vi "Extended Kalman Filter (GPS & IMU Fusion) 수정중(H=eye(4)로).vi"(0 "R (v의 공분산행렬_측정잡음)_모델링필요":dbl[][](array[numeric])=[[100000000.0, 0.0, 0.0, 0.0], [0.0, 100000000.0, 0.0, 0.0], [0.0, 0.0, 100000.0, 0.0], [0.0, 0.0, 0.0, 10.0]], 4 "Q (w의 공분산행렬_시스템잡음)_모델링필요":dbl[][](array[numeric])=[[50000.0, 0.0, 0.0, 0.0], [0.0, 50000.0, 0.0, 0.0], [0.0, 0.0, 0.001, 0.0], [0.0, 0.0, 0.0, 0.01]], 5 "theta_IMU":dbl, 6 "dt (측정주기)":dbl=0.02, 7 "v_Encoder":dbl, 10 "X_GPS Raw":dbl[](array[numeric])) -> (2 "X_EKF":dbl[](array[numeric]))   [LabVIEW 2016]
uses:
  <vilib>/imath/engines/lvmath2/RunTimeEngine/IndexRead/NIMS M(S).vi
  <instcachedir>/0/NIMS M(S)_B826C018497E4940AE96BD27B540B6FB.lvgen/NIMS M(S)_B826C018497E4940AE96BD27B540B6FB_000.vi
  <vilib>/imathl/engines/lvmath/Functions/Error Handling/Create Error.vi
  <vilib>/imath/engines/lvmath2/RunTimeEngine/BuiltInFunctions/deg_to_rad/NIMS_deg_to_rad.vi
  <instcachedir>/0/NIMS_deg_to_rad_4A81D684CE8D4DD79924F5AB74D756E1.lvgen/NIMS_deg_to_rad_4A81D684CE8D4DD79924F5AB74D756E1_001.vi
  <vilib>/imath/engines/lvmath2/RunTimeEngine/ArithmeticOperatorToken/NIMS_ArithmeticOperator_multmx.vi
  <instcachedir>/0/NIMS_ArithmeticOperator_multmx_4A56FE5C615140CE835D4DB5891BF065.lvgen/NIMS_ArithmeticOperator_multmx_4A56FE5C615140CE835D4DB5891BF065_004.vi
  <vilib>/imath/engines/lvmath2/RunTimeEngine/ArithmeticOperatorToken/NIMS_ArithmeticOperator_plus.vi
  <instcachedir>/0/NIMS_ArithmeticOperator_plus_0120E0498A0F4B4B9BDCAC2554767A4E.lvgen/NIMS_ArithmeticOperator_plus_0120E0498A0F4B4B9BDCAC2554767A4E_003.vi
  <vilib>/imath/engines/lvmath2/RunTimeEngine/ErrorHandling/NIMS_Create Error From Enums.vi
  <vilib>/imath/engines/lvmath2/RunTimeEngine/BuiltInFunctions/inv/NIMS_inv(GM).vi
  <instcachedir>/0/NIMS_inv(GM)_A6DF8FE880224208AACFE4CF9F659502.lvgen/NIMS_inv(GM)_A6DF8FE880224208AACFE4CF9F659502_000.vi
  <vilib>/imath/engines/lvmath2/RunTimeEngine/ArithmeticOperatorToken/NIMS_ArithmeticOperator_multmx(M,CV).vi
  <instcachedir>/0/NIMS_ArithmeticOperator_multmx(M,CV)_EE734FC8520844C9A7CC1A67008668A3.lvgen/NIMS_ArithmeticOperator_multmx(M,CV)_EE734FC8520844C9A7CC1A67008668A3_000.vi
  <vilib>/imath/engines/lvmath2/RunTimeEngine/ArithmeticOperatorToken/NIMS_ArithmeticOperator_minus.vi
  <instcachedir>/0/NIMS_ArithmeticOperator_minus_E3B65B1D26A44BB184AFDC5B3F458E3D.lvgen/NIMS_ArithmeticOperator_minus_E3B65B1D26A44BB184AFDC5B3F458E3D_002.vi
  <vilib>/imath/engines/lvmath2/RunTimeEngine/NodeEndStatement/NIMS_NodeEndStatement_Output.vi
  <instcachedir>/0/NIMS_NodeEndStatement_Output_53EC0D466D134D7ABD903AC30B43404B.lvgen/NIMS_NodeEndStatement_Output_53EC0D466D134D7ABD903AC30B43404B_002.vi
  <vilib>/imath/engines/lvmath2/RunTimeEngine/ErrorHandling/NIMS_Finalize Error.vi
panel:
  out "P (Covariance Matrix))":dbl[][](array[numeric])
  out "K (Kalman Gain)":dbl[][](array[numeric])
  in  "P0 (공분산 행렬 초기값)_모델링필요":dbl[][](array[numeric])=[[1.0, 0.0, 0.0, 0.0], [0.0, 1.0, 0.0, 0.0], [0.0, 0.0, 1.0, 0.0], [0.0, 0.0, 0.0, 1.0]]
  # "GPS 측정값\n \n  GPS Input = [ x_Nav  y_Nav  h  theta_GPS ]'\n\n      x_Nav : 항법좌표계로 변환한 X좌표\n\n      y_Nav : 항법좌표계로 변환한 Y좌표\n\n      theta_GPS : 방향각 (Heading angle)\n\n      v_GPS: 차량의 속도 (Speed)"
  # "X(State)= [ x y theta v ]'"
  # "IMU & Encoder 측정값\n\n       theta_IMU : 방향각 (yaw angle)\n\n       v_Encoder : 차량의 속도 (Speed)"
  # "모델링 필요\n\n1, X0:   상태변수 초기값\n2. dt:    측정시간 (Hz)\n2. P0:   공분산행렬 초기값\n3. Q:    시스템노이즈 공분산행렬\n4. R:     측정노이즈 공분산행렬"
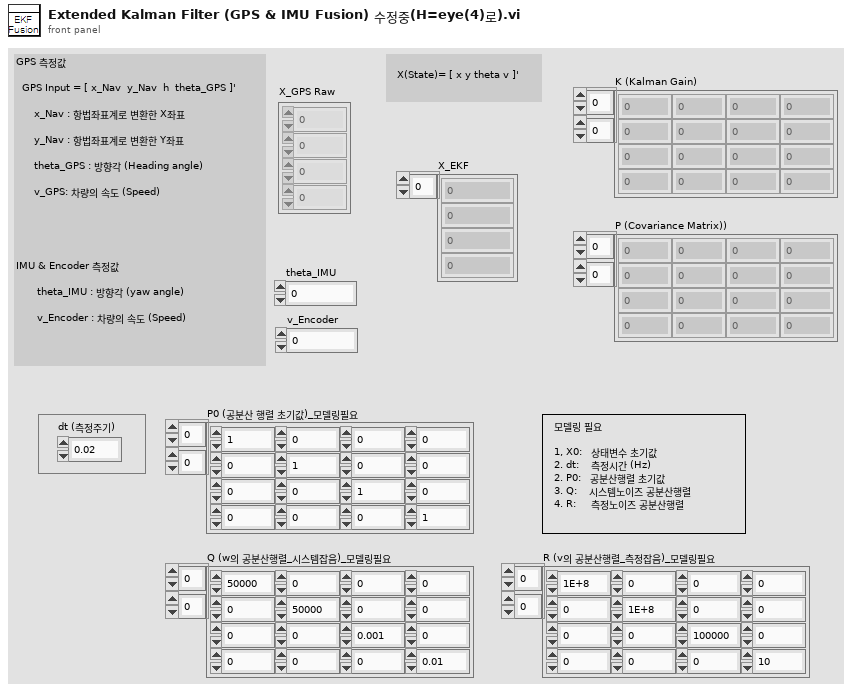
[diagram p1: front panel]
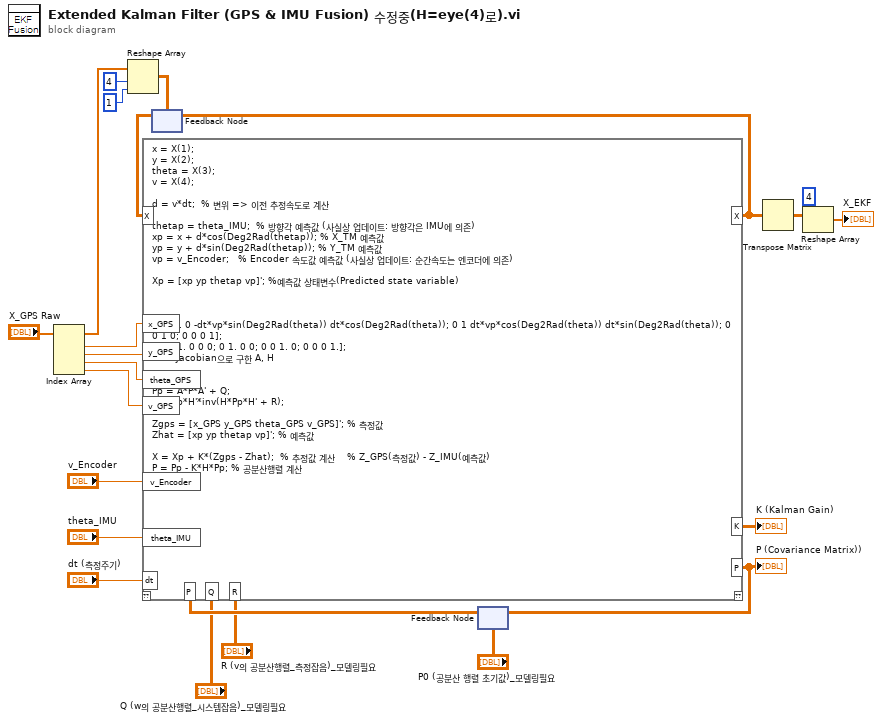
[diagram p0: block diagram]
diagram:
  n1 = Index Array(array="X_GPS Raw") -> (element #1=w9:dbl, element #2=w7:dbl, element #3=w6:dbl, element #4=w8:dbl)  [unwired: 4 in]
  n2 = Reshape Array("X_GPS Raw", 4 ("차원 크기"), 1 ("차원 크기")) -> (w12:dbl[][])
  n3 = feedback #1(w12) -> (w15:dbl[][])
  n4 = feedback #2("P0 (공분산 행렬 초기값)_모델링필요") -> (w21:dbl[][])
  n5 = mathscript code="x = X(1);\ny = X(2);\ntheta = X(3);\nv = X(4);\n\nd = v*dt;  % 변위 => 이전 추정속도로 계산\n\nthetap = theta_IMU;  % 방향각 예측값 (사실상 업데이트: 방향각은 IMU에 의존)\nxp = x + d*cos(Deg2Rad(thetap)); % X_TM 예측값\nyp = y + d*sin(Deg2Rad(thetap)); % Y_TM 예측값\nvp = v_Encoder;   % Encoder 속도값 예측값 (사실상 업데이트: 순간속도는 엔코더에 의존)\n\nXp = [xp yp thetap vp]'; %예측값 상태변수(Predicted state variable)\n\n\n\nA = [1 0 -dt*vp*sin(Deg2Rad(theta)) dt*cos(Deg2Rad(theta)); 0 1 dt*vp*cos(Deg2Rad(theta)) dt*sin(Deg2Rad(theta)); 0 0 1 0; 0 0 0 1];\nH = [1. 0 0 0; 0 1. 0 0; 0 0 1. 0; 0 0 0 1.];\n%%  Jacobian으로 구한 A, H\n\n\nPp = A*P*A' + Q;\nK = Pp*H'*inv(H*Pp*H' + R);\n\nZgps = [x_GPS y_GPS theta_GPS v_GPS]'; % 측정값\nZhat = [xp yp thetap vp]'; % 예측값\n\nX = Xp + K*(Zgps - Zhat);  % 추정값 계산    % Z_GPS(측정값) - Z_IMU(예측값)\nP = Pp - K*H*Pp; % 공분산행렬 계산"("dt"="dt (측정주기)", "v_Encoder"="v_Encoder", "P"=w21, "Q"="Q (w의 공분산행렬_시스템잡음)_모델링필요", "R"="R (v의 공분산행렬_측정잡음)_모델링필요", "x_GPS"=w9, "y_GPS"=w7, "theta_GPS"=w6, "theta_IMU"="theta_IMU", "X"=w15, "v_GPS"=w8) -> ("X"=w2:dbl[][], "P"=w22:dbl[][], "K"=→"K (Kalman Gain)":dbl[][])  [unwired: 1 in, 1 out]
  "P (Covariance Matrix))" <- w22
  n6 = feedback-in #1(w2) -> ()
  n7 = feedback-in #2(w22) -> ()
  n8 = Transpose Matrix ("전치 행렬")(1:w2) -> (0:w3:dbl[][])
  n9 = Reshape Array ("배열 차원 변경")(w3, 4 ("차원 크기")) -> (→"X_EKF":dbl[])
